vi "test Dequeue Timeout.vi"(8 "error in (no error)":errorcluster, 11 "TestCase in":refnum<class "Message Queue Test Case.lvclass">) -> (0 "error out":errorcluster, 3 "TestCase out":refnum<class "Message Queue Test Case.lvclass">)   [LabVIEW 2027, in "Message Queue Test Case.lvclass"]
uses:
  Message Queue Test Case.lvclass
  Message/Abstract Message/Abstract Message.lvclass
  Message Queue Test Case.lvclass/Message Queue Test Case.ctl
  Message Queue/Abstract Message Queue/Abstract Message Queue.lvclass
  C:/Program Files/National Instruments/LabVIEW 2027/vi.lib/addons/_JKI Toolkits/VI Tester/TestCase.llb/TestCase.lvclass
  <vilib>/addons/_JKI Toolkits/VI Tester/TestCase.llb/TestCase.lvclass
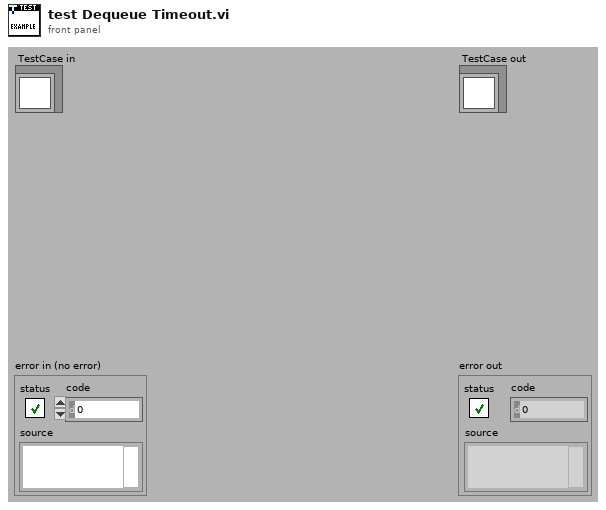
[diagram p1: front panel]
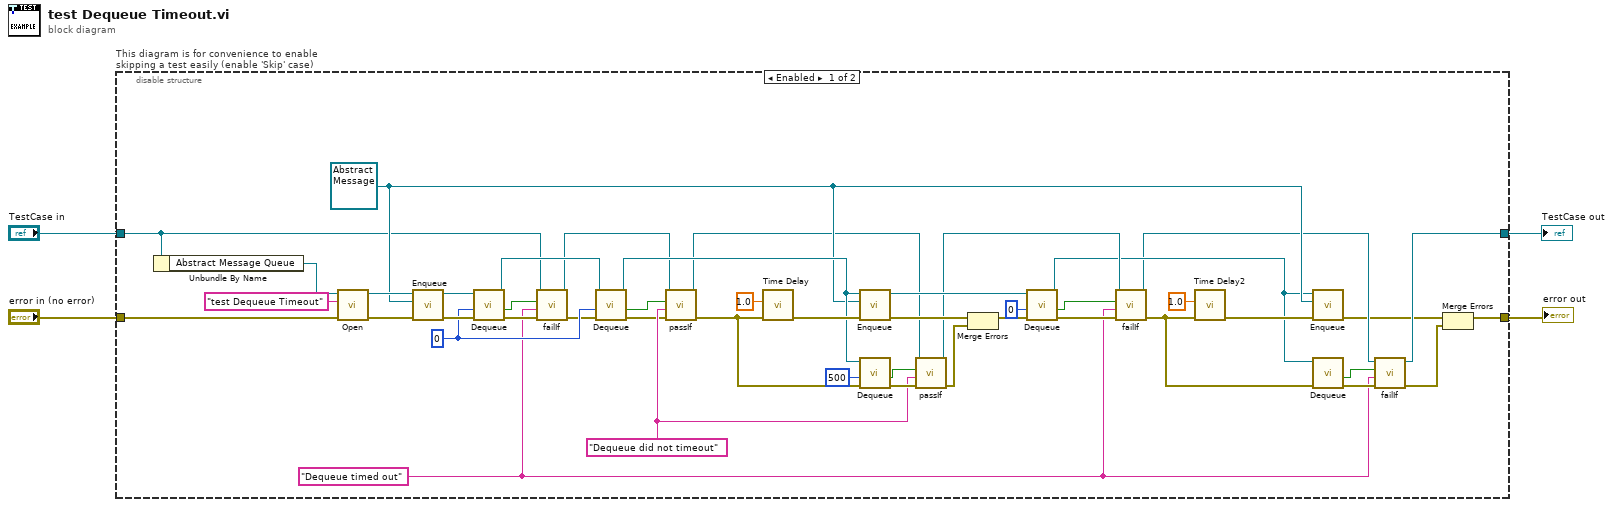
[diagram p0: block diagram]
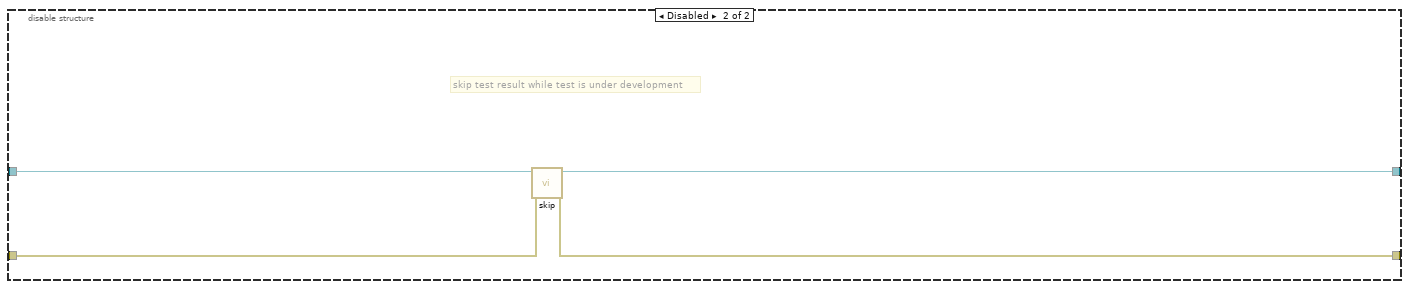
[diagram p2: hidden frame]
diagram:
  n1 = disable-structure "This diagram is for convenience to enable skipping a test easily (enable 'Skip' case)" shown="Enabled" {
    disable-tunnel: "TestCase in" -> [w26 w54]
    disable-tunnel: [w12 w52] -> w1
    disable-tunnel: [w9 w53] -> w3
    disable-tunnel: "error in (no error)" -> [w50 w51]
    frame Enabled {
      w14 = "Dequeue timed out" ("message (\"\")")
      w35 = "Dequeue did not timeout" ("message (\"\")")
      w42 = 0 ("timeout in ms (-1)")
      w28 = refnum<class "Abstract Message.lvclass"> refnum ("Message in")
      n2 = Unbundle By Name(w26) -> ("Abstract Message Queue"=w49:refnum<class "Abstract Message Queue.lvclass">)
      n3 = call-dynamic "Open.vi"("error in (no error)"=w50, "name (unnamed)"="test Dequeue Timeout", "Abstract Message Queue in"=w49) -> ("error out"=w47:errorcluster, "Abstract Message Queue out"=w46:refnum<class "Abstract Message Queue.lvclass">)  [unwired: 7 in]
      n4 = call-dynamic "Enqueue.vi"("error in (no error)"=w47, "Message in"=w28, "Abstract Message Queue in"=w46) -> ("error out"=w45:errorcluster, "Abstract Message Queue out"=w44:refnum<class "Abstract Message Queue.lvclass">)  [unwired: 7 in]
      n5 = call-dynamic "Dequeue.vi"("error in (no error)"=w45, "timeout in ms (-1)"=w42, "Abstract Message Queue in"=w44) -> ("error out"=w27:errorcluster, "timed out?"=w19:bool, "Abstract Message Queue out"=w43:refnum<class "Abstract Message Queue.lvclass">)  [unwired: 5 in, 1 out]
      n6 = call-dynamic "failIf.vi"("error in (no error)"=w27, "message (\"\")"=w14, "fail"=w19, "TestCase in"=w26) -> ("error out"=w8:errorcluster, "TestCase out"=w25:refnum<class "Message Queue Test Case.lvclass">)  [unwired: 6 in]
      n7 = call-dynamic "Dequeue.vi"("error in (no error)"=w8, "timeout in ms (-1)"=w42, "Abstract Message Queue in"=w43) -> ("error out"=w7:errorcluster, "timed out?"=w41:bool, "Abstract Message Queue out"=w34:refnum<class "Abstract Message Queue.lvclass">)  [unwired: 5 in, 1 out]
      n8 = call-dynamic "passIf.vi"("error in (no error)"=w7, "message (\"\")"=w35, "pass"=w41, "TestCase in"=w25) -> ("error out"=w39:errorcluster, "TestCase out"=w22:refnum<class "Message Queue Test Case.lvclass">)  [unwired: 6 in]
      n9 = call "Time Delay"("error in (no error)"=w39, "Delay Time (s)"=1.0) -> ("error out"=w38:errorcluster)  [unwired: 9 in]
      n10 = call-dynamic "Enqueue.vi"("error in (no error)"=w38, "Message in"=w28, "Abstract Message Queue in"=w34) -> ("error out"=w32:errorcluster, "Abstract Message Queue out"=w30:refnum<class "Abstract Message Queue.lvclass">)  [unwired: 7 in]
      n11 = call-dynamic "Dequeue.vi"("error in (no error)"=w39, "timeout in ms (-1)"=500, "Abstract Message Queue in"=w34) -> ("error out"=w37:errorcluster, "timed out?"=w36:bool)  [unwired: 5 in, 2 out]
      n12 = call-dynamic "passIf.vi"("error in (no error)"=w37, "message (\"\")"=w35, "pass"=w36, "TestCase in"=w22) -> ("error out"=w6:errorcluster, "TestCase out"=w21:refnum<class "Message Queue Test Case.lvclass">)  [unwired: 6 in]
      n13 = Merge Errors(w32, w6) -> (w31:errorcluster)
      n14 = call-dynamic "Dequeue.vi"("error in (no error)"=w31, "timeout in ms (-1)"=0, "Abstract Message Queue in"=w30) -> ("error out"=w23:errorcluster, "timed out?"=w18:bool, "Abstract Message Queue out"=w16:refnum<class "Abstract Message Queue.lvclass">)  [unwired: 5 in, 1 out]
      n15 = call-dynamic "failIf.vi"("error in (no error)"=w23, "message (\"\")"=w14, "fail"=w18, "TestCase in"=w21) -> ("error out"=w20:errorcluster, "TestCase out"=w13:refnum<class "Message Queue Test Case.lvclass">)  [unwired: 6 in]
      n16 = call "Time Delay2"("error in (no error)"=w20, "Delay Time (s)"=1.0) -> ("error out"=w24:errorcluster)  [unwired: 9 in]
      n17 = call-dynamic "Enqueue.vi"("error in (no error)"=w24, "Message in"=w28, "Abstract Message Queue in"=w16) -> ("error out"=w11:errorcluster)  [unwired: 7 in, 1 out]
      n18 = call-dynamic "Dequeue.vi"("error in (no error)"=w20, "Abstract Message Queue in"=w16) -> ("error out"=w17:errorcluster, "timed out?"=w15:bool)  [unwired: 6 in, 2 out]
      n19 = call-dynamic "failIf.vi"("error in (no error)"=w17, "message (\"\")"=w14, "fail"=w15, "TestCase in"=w13) -> ("error out"=w10:errorcluster, "TestCase out"=w12:refnum<class "Message Queue Test Case.lvclass">)  [unwired: 6 in]
      n20 = Merge Errors(w11, w10) -> (w9:errorcluster)
    }
    frame Disabled {
      # "skip test result while test is under development"
      n21 = call <vilib>:"skip.vi"("error in (no error)"=w51, "TestCase in"=w54) -> ("error out"=w53:errorcluster, "TestCase out"=w52:refnum<class "Message Queue Test Case.lvclass">)  [unwired: 8 in]
    }
  }
  "error out" <- w3
  "TestCase out" <- w1
